vi "Wait for Deposit.vi"(8 "error in":errorcluster, 11 "Account info":T1) -> (0 "error out":errorcluster, 1 "Stop?":bool, 2 "Deposit Amount":dbl, 3 "Account info out":T1)   [LabVIEW 2012]
uses:
  Account Info.ctl
  Stop.vi
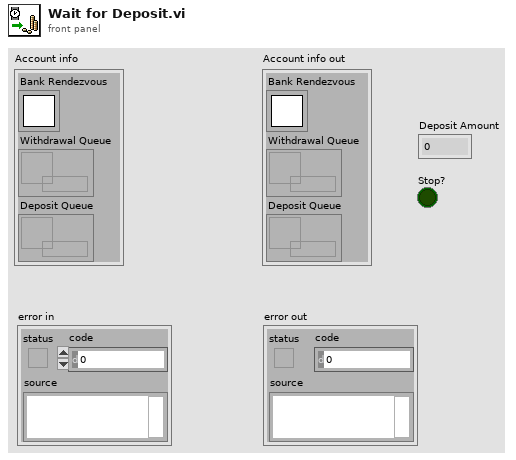
[diagram p1: front panel]
types:
  T1 = typedef "Account Info.ctl" = cluster{"Bank Rendezvous":T2, "Withdrawal Queue":refnum<queue>, "Deposit Queue":refnum<queue>}
  T2 = typedef "Rendezvous RefNum" = refnum<k1>
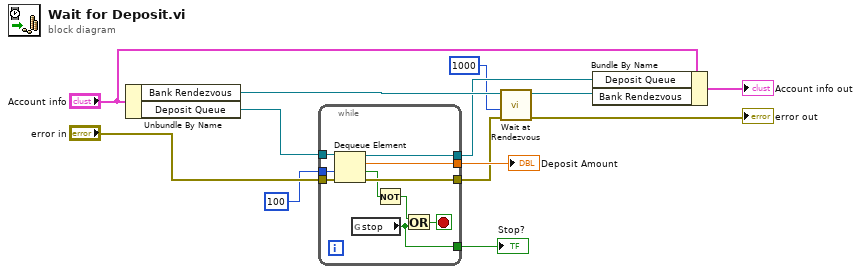
[diagram p0: block diagram]
diagram:
  n1 = Unbundle By Name("Account info") -> ("Bank Rendezvous"=w10:T2, "Deposit Queue"=w13:refnum<queue>)
  n2 = while {
    tunnel: w13 -> [w23]
    tunnel: [w22] -> w12
    tunnel: "error in" -> [w21]
    tunnel: [w20] -> w9
    tunnel: [w19] -> w6
    tunnel: 100 ("timeout in ms (-1)") -> [w15]
    tunnel: [w14] -> w1
    stop <- w18 stop-if-true
    n3 = Dequeue Element(queue=w23, timeout in ms (-1)=w15, error in (no error)=w21) -> (queue out=w19:refnum<queue>, element=w22:dbl, timed out?=w16:bool, error out=w20:errorcluster)
    n4 = global read "Stop.vi" "stop"() -> (w14:bool)
    n5 = Not(x=w16) -> (.not. x?=w17:bool)
    n6 = Or(x=w17, y=w14) -> (x .or. y?=w18:bool)
  }
  "Deposit Amount" <- w12
  "Stop?" <- w1
  n7 = call <vilib>:"Wait at Rendezvous.vi"("error in (no error)"=w9, "ms timeout (-1)"=1000, "rendezvous"=w10) -> ("error out"=→"error out":errorcluster, "rendezvous out"=w7:T2)  [unwired: 2 in, 1 out]
  n8 = Bundle By Name(cluster="Account info", "Deposit Queue"=w6, "Bank Rendezvous"=w7) -> (→"Account info out":T1)
